vi "TEST_MoveRectangle.vi"() -> ()   [LabVIEW 2021, in "Picture2D.lvlib"]
uses:
  Picture2D/Picture2D.lvlib
  Rectangle/Rectangle.lvclass
  C:/GitHub/Picture2D/src/Shape/Shape.lvclass
  Color/Color.lvclass
  Pen/Pen.lvclass
  PointSpecialized/PointSpecialized.lvclass
  C:/GitHub/Picture2D/src/Point/Point.lvclass
panel:
  in  "Point:StartPoint":cluster{"x":i16, "y":i16}={"x"=-10, "y"=-10}
  in  "Point:ToMove":cluster{"x":i16, "y":i16}={"x"=-10, "y"=-10}
  in  "Pen:Style":T1(ring)
  in  "Pen:Width":u16=10
  in  "Absolute":bool
  out "2D Picture":picture
  in  "Color Box":u32(colorbox)=16711680
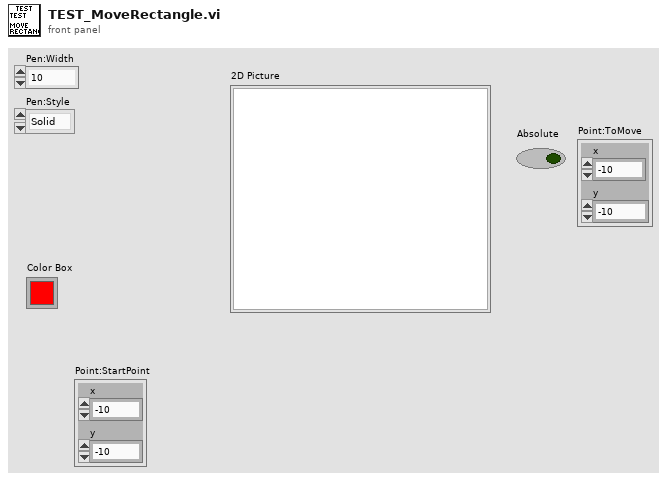
[diagram p1: front panel]
types:
  T1 = enum32{"Solid", "Dash", "Dot", "DashDot", "DashDotDot"}
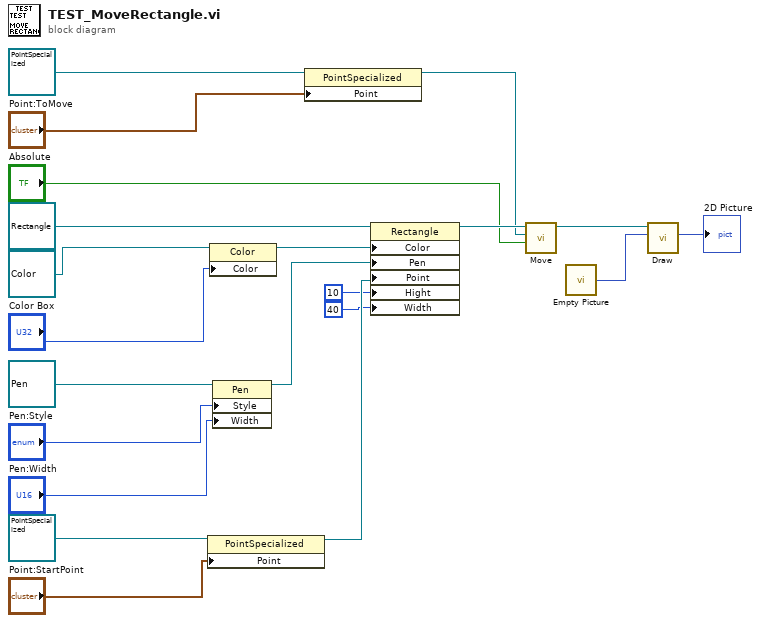
[diagram p0: block diagram]
diagram:
  n1 = property class="PointSpecialized"(reference=refnum<class "PointSpecialized.lvclass"> refnum ("Point"), "Point"="Point:StartPoint") -> (reference out=w3:refnum<class "PointSpecialized.lvclass">)  [unwired: 1 in, 1 out]
  n2 = property class="Color"(reference=refnum<class "Color.lvclass"> refnum ("Color"), "Color"="Color Box") -> (reference out=w20:refnum<class "Color.lvclass">)  [unwired: 1 in, 1 out]
  n3 = property class="Pen"(reference=refnum<class "Pen.lvclass"> refnum ("Pen"), "Style"="Pen:Style", "Width"="Pen:Width") -> (reference out=w16:refnum<class "Pen.lvclass">)  [unwired: 1 in, 1 out]
  n4 = property class="PointSpecialized"(reference=refnum<class "PointSpecialized.lvclass"> refnum ("Point"), "Point"="Point:ToMove") -> (reference out=w7:refnum<class "PointSpecialized.lvclass">)  [unwired: 1 in, 1 out]
  n5 = property class="Rectangle"(reference=refnum<class "Rectangle.lvclass"> refnum ("Rectangle"), "Color"=w20, "Pen"=w16, "Point"=w3, "Hight"=i16 10, "Width"=i16 40) -> (reference out=w11:refnum<class "Rectangle.lvclass">)  [unwired: 1 in, 1 out]
  n6 = call-dynamic "Move.vi"("Absolute (T)"="Absolute", "Point"=w7, "Rectangle in"=w11) -> ("Rectangle out"=w10:refnum<class "Rectangle.lvclass">)  [unwired: 7 in, 1 out]
  n7 = call "Empty Picture"() -> ("empty picture"=w13:picture)
  n8 = call-dynamic "Draw.vi"("2D Picture in"=w13, "Rectangle in"=w10) -> ("2D Picture out"=→"2D Picture":picture)  [unwired: 7 in, 2 out]
